vi "Set Unsaved Changes in Title.vi"(7 "VI in":refnum<vi>, 10 "error in (no error)":errorcluster, 11 "Unsaved changes? (F)":bool) -> (2 "error out":errorcluster)   [LabVIEW 2020, in "RxnRover.lvlib"]
doc: "Update the Reaction Rover window title to have an asterisk (*) after the project file location, indicating that there are unsaved changes to the project."
uses:
  RxnRover.lvlib
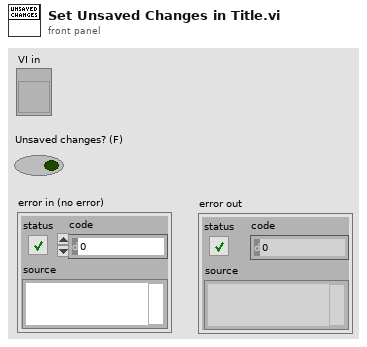
[diagram p1: front panel]
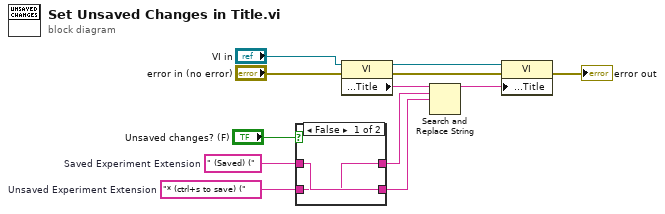
[diagram p0: block diagram]
diagram:
  w4 = "* (ctrl+s to save) ("  # Unsaved Experiment Extension
  w5 = " (Saved) ("  # Saved Experiment Extension
  n1 = case shown="False" "Unsaved changes? (F)" {
    tunnel: w5 -> [w14 w16]
    tunnel: w4 -> [w13 w15]
    tunnel: [w13 w16] -> w3
    tunnel: [w14 w15] -> w2
    frame False {
    }
    frame True {
    }
  }
  n2 = property class="VI"(reference="VI in", error in="error in (no error)") -> (reference out=w9:refnum<vi>, error out=w1:errorcluster, "Front Panel.Title"=w8:string)
  n3 = Search and Replace String(input string=w8, search string=w3, replace string=w2) -> (result string=w7:string)  [unwired: 5 in, 3 out]
  n4 = property class="VI"(reference=w9, error in=w1, "Front Panel.Title"=w7) -> (error out=→"error out":errorcluster)  [unwired: 1 out]
